vi "ConnectDev.vi"(1 "IP.":string caption="IP地址") -> (0 "connection ID":refnum<k5>)   [LabVIEW 2012]
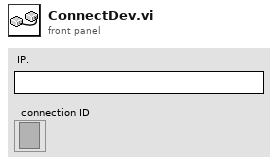
[diagram p1: front panel]
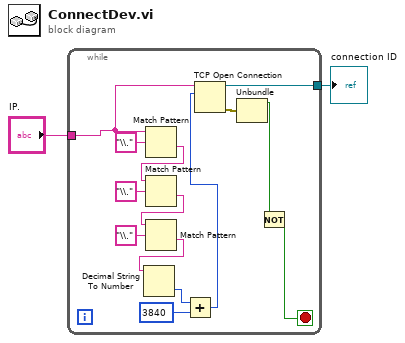
[diagram p0: block diagram]
diagram:
  n1 = while {
    tunnel: [w16] -> w1
    tunnel: "IP." -> [w15]
    stop <- w3 stop-if-true
    n2 = Match Pattern(string=w15, regular expression="\\." ("正则表达式")) -> (after substring=w11:string)  [unwired: 1 in, 3 out]
    n3 = Match Pattern(string=w11, regular expression="\\." ("正则表达式")) -> (after substring=w10:string)  [unwired: 1 in, 3 out]
    n4 = Match Pattern(string=w10, regular expression="\\." ("正则表达式")) -> (after substring=w9:string)  [unwired: 1 in, 3 out]
    n5 = Decimal String To Number(string=w9) -> (number=w8:i32)  [unwired: 2 in, 1 out]
    n6 = Add(x=w8, y=3840) -> (x+y=w6:i32)
    n7 = TCP Open Connection(address=w15, remote port or service name=w6) -> (connection ID=w16:refnum<k5>, error out=w5:errorcluster)  [unwired: 3 in]
    n8 = Unbundle(w5) -> ("status"=w4:bool)  [unwired: 2 out]
    n9 = Not(x=w4) -> (.not. x?=w3:bool)
  }
  "connection ID" <- w1
